vi "HeaderBlock.vi"(8 "error in (no error)":errorcluster, 11 "Head":cluster{"Title":string, "Created":string}) -> (0 "error out":errorcluster, 3 "Header Block Out":string)   [LabVIEW 2016]
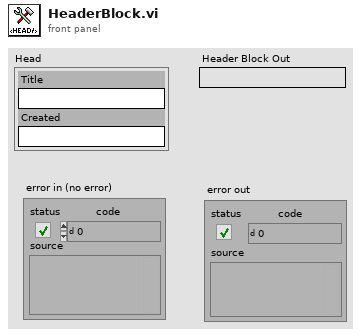
[diagram p1: front panel]
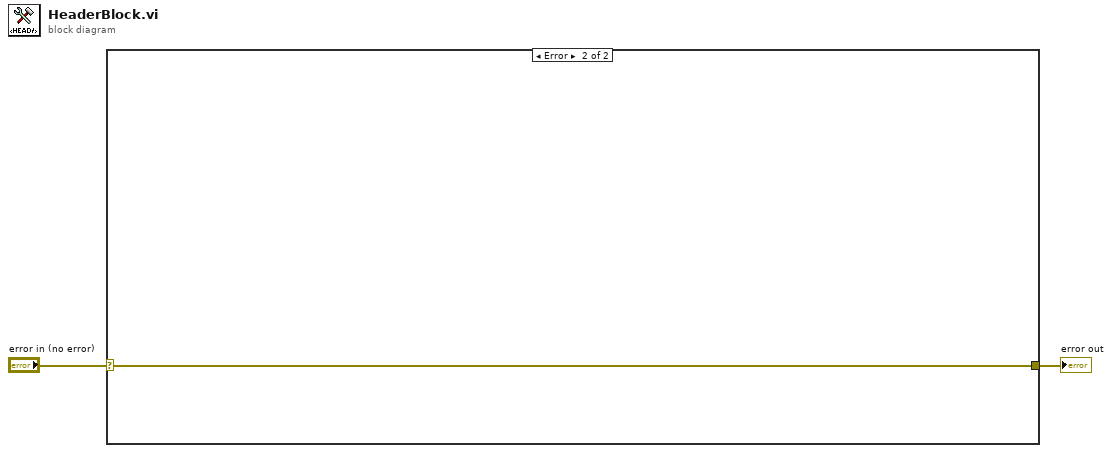
[diagram p0: block diagram]
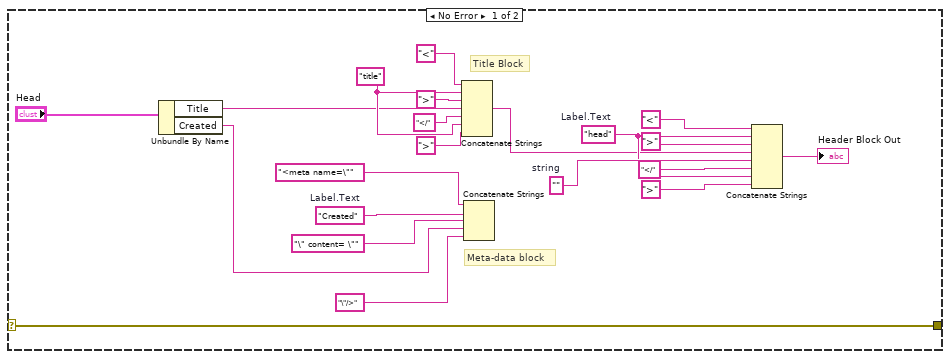
[diagram p2: hidden frame]
diagram:
  n1 = case shown="Error" "error in (no error)" {
    selector: "error in (no error)" -> [w3 w24]
    tunnel: [w3 w24] -> w1
    frame No Error {
      w23 = ""  # string
      w22 = "head"  # Label.Text
      w21 = "title"
      w20 = "Created"  # Label.Text
      # "Meta-data block"
      # "Title Block"
      n2 = Unbundle By Name("Head") -> ("Title"=w8:string, "Created"=w14:string)
      n3 = Concatenate Strings("<" ("string"), w21, ">" ("string"), w8, "</" ("string"), w21, ">" ("string")) -> (w13:string)
      n4 = Concatenate Strings("<meta name=\"" ("string"), w20, "\" content= \"" ("string"), w14, "\"/>" ("string")) -> ()  [unwired: 1 out]
      n5 = Concatenate Strings("<" ("string"), w22, ">" ("string"), w13, w23, "</" ("string"), w22, ">" ("string")) -> (→"Header Block Out":string)
    }
    frame Error {
    }
  }
  "error out" <- w1
